vi "Example - All Devices.vi"() -> ()   [LabVIEW 2022 SP3]
uses:
  Logitech Devices/Logitech Devices.lvlib
  Logitech Devices/Public/TypeDefs/Speaker Lighting Zones.ctl
  Logitech Devices/Public/TypeDefs/Mouse Lighting Zones.ctl
panel:
  out "error out":errorcluster
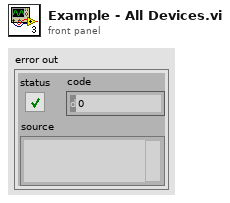
[diagram p1: front panel]
types:
  T1 = typedef "Logitech Devices.lvlib/Mouse Lighting Zones.ctl" = enum8{"DPI Indicator", "Logo"}
  T2 = typedef "Logitech Devices.lvlib/Speaker Lighting Zones.ctl" = enum8{"Front left", "Front right", "Rear left", "Rear right"}
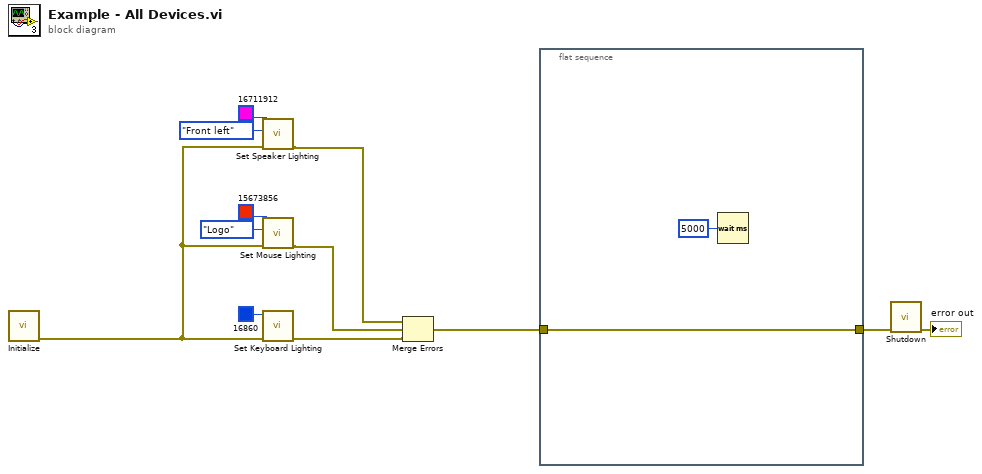
[diagram p0: block diagram]
diagram:
  n1 = call "Initialize.vi"() -> ("error out"=w7:errorcluster)  [unwired: 11 in]
  n2 = call "Set Speaker Lighting.vi"("error in (no error)"=w7, "Lighting Zone"=Speaker_Lighting_Zones."Front left", "LED Color"=u32 16711912) -> ("error out"=w5:errorcluster)  [unwired: 8 in]
  n3 = call "Set Mouse Lighting.vi"("error in (no error)"=w7, "Lighting Zone"=Mouse_Lighting_Zones."Logo", "LED Color"=u32 15673856) -> ("error out"=w4:errorcluster)  [unwired: 8 in]
  n4 = call "Set Keyboard Lighting.vi"("error in (no error)"=w7, "LED Color"=u32 16860) -> ("error out"=w6:errorcluster)  [unwired: 9 in]
  n5 = Merge Errors(w5, w4, w6) -> (w3:errorcluster)
  n6 = flat-sequence {
    tunnel: w3 -> [w13]
    tunnel: [w13] -> w2
    frame #0 {
      n7 = Wait (ms)(milliseconds to wait=u32 5000) -> ()  [unwired: 1 out]
    }
  }
  n8 = call "Shutdown.vi"("error in (no error)"=w2) -> ("error out"=→"error out":errorcluster)  [unwired: 10 in]
